vi "VisionV4 2-12-20.vi"(0 "Range (Threshold 1)":cluster{"Lower value":sgl, "Upper value":sgl}={"Lower value"=210.0, "Upper value"=250.0}, 1 "Minimal Score (Shape Matching 1)":dbl=400.0, 2 "Scale Invariance (Shape Matching 1)":bool=TRUE, 3 "Image":T1(plugin-control), 7 "error in":errorcluster) -> (20 "Histogram (Histogram 1)":u32[][](array[numeric]), 21 "Statistics (Histogram 1)":T3 {"Standard  Variation" format="%.2f"; "Mean Value" format="%.2f"; "Maximal Value" format="%.2f"; "Minimal Value" format="%.2f"}, 22 "Number of Matches (Shape Matching 1)":i32, 23 "Shape Report (Shape Matching 1)":T2(array[cluster]) {"Score" format="%.2f"; "Centroid"."y" format="%.2f"; "Centroid"."x" format="%.2f"}, 27 "error out":errorcluster)   [LabVIEW 2019]
uses:
  <vilib>/vision/NI_Vision_Development_Module.lvlib
panel:
  out "Image Out":T1(plugin-control)
  out "Histogram Graph":u32[][](graph)
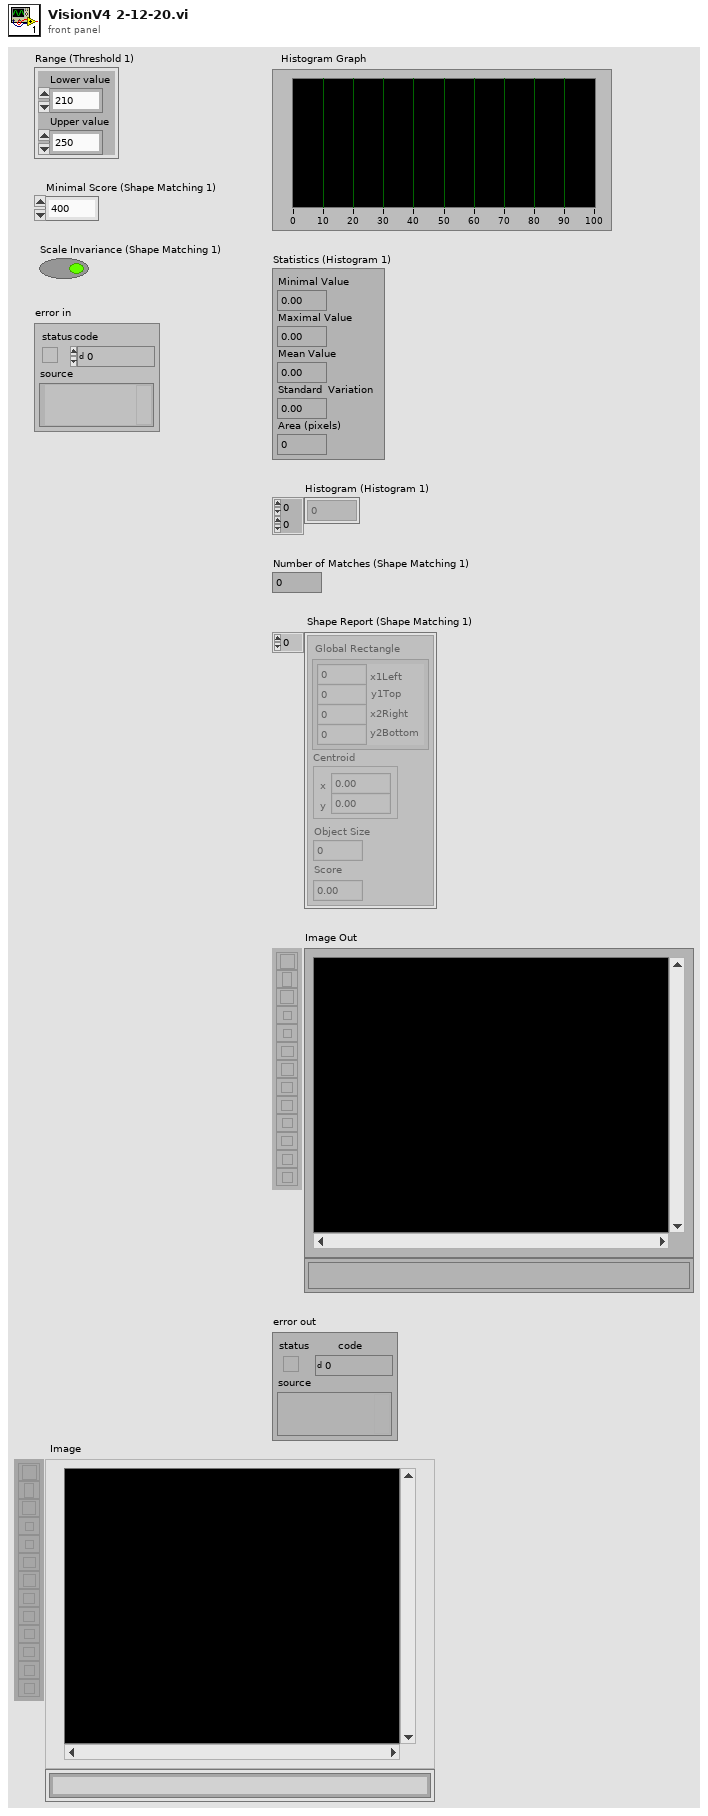
[diagram p1: front panel]
types:
  T1 = typedef "IMAQ Image.ctl" = refnum<image>
  T2 = cluster{"Global Rectangle":cluster{"x1Left":i32, "y1Top":i32, "x2Right":i32, "y2Bottom":i32}, "Centroid":cluster{"x":sgl, "y":sgl}, "Object Size":u32, "Score":dbl}[]
  T3 = cluster{"Minimal Value":sgl, "Maximal Value":sgl, "Mean Value":sgl, "Standard  Variation":sgl, "Area (pixels)":i32}
  T4 = cluster{"Measurement Parameter":i32, "Range Lower Value":dbl, "Range Upper Value":dbl, "Range":bool, "Measurement Type":bool}[]
  T5 = cluster{"Global Rectangle":i32[], "Contours":cluster{"ID":enum32{"External", "Internal"}, "Type":u32, "Coordinates":i32[]}[]}
  T6 = cluster{"histogram":u32[], "Minimal Value":sgl, "Maximal Value":sgl, "Starting Value":sgl, "Interval Width":sgl, "Mean Value":sgl, "Standard  Variation":sgl, "Area (pixels)":i32}
  T7 = typedef "Image Type" = u32
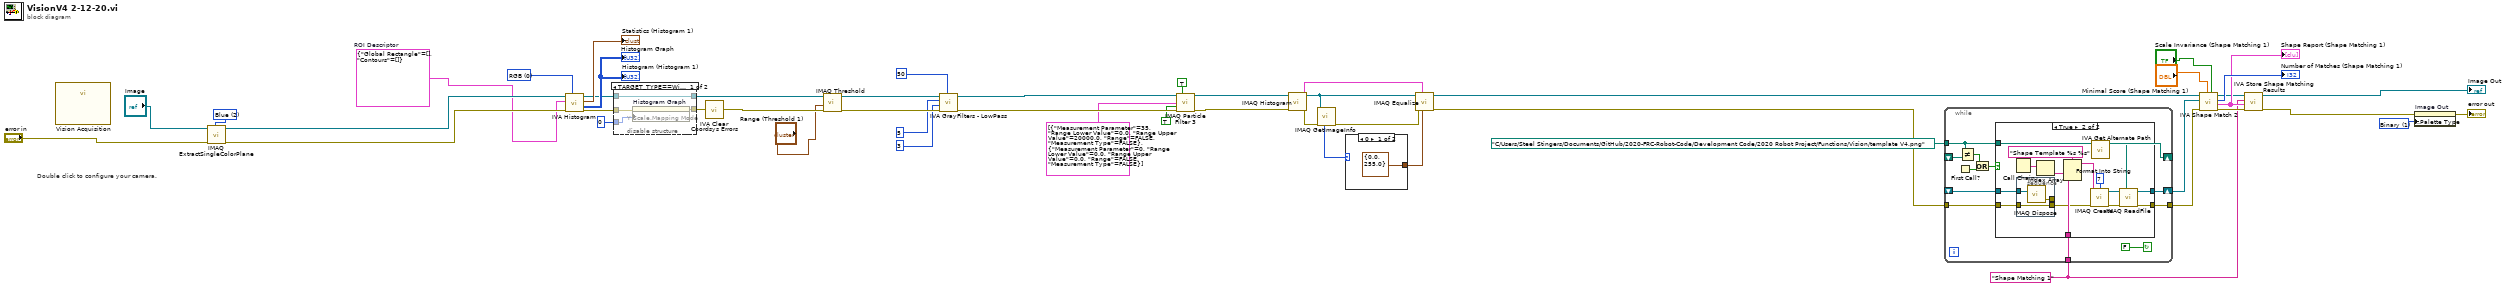
[diagram p0: block diagram]
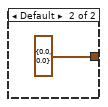
[diagram p3: hidden frame]
diagram:
  w3 = u32 1 items=["Grayscale", "Binary", "Gradient", "Rainbow", "Temperature", "User Defined", "Binary 16 Bit", "Gradient 16 Bit", "Rainbow 16 Bit", "Temperature 16 Bit", "User Defined 16 Bit"] ("Palette Type")
  w6 = "Shape Matching 1" ("Step Name")
  w44 = u16 0 items=["RGB", "HSL", "HSV", "HSI"] ("Color Mode")
  w42 = T5 {"Global Rectangle"=[], "Contours"=[]}  # ROI Descriptor
  w49 = 2 items=["Red", "Green", "Blue", "Hue", "Saturation", "Luminance", "Value", "Intensity"] ("Color Plane")
  # "Double click to configure your camera."
  n1 = call "Vision Acquisition"() -> ()  [unwired: 20 in]
  n2 = call "IMAQ ExtractSingleColorPlane"("Color Plane"=w49, "error in (no error)"="error in", "Image Src"="Image") -> ("error out"=w48:errorcluster, "Image Dst Out"=w47:T1)  [unwired: 1 in, 6 out]
  n3 = call <vilib>:"IVA Histogram.vi"("Color Mode"=w44, "error in (no error)"=w48, "ROI Descriptor"=w42, "Image In"=w47) -> ("error out"=w45:errorcluster, "Histograms"=→"Histogram Graph" →"Histogram (Histogram 1)":u32[][], "Statistics"=→"Statistics (Histogram 1)":T3, "Image Out"=w41:T1)  [unwired: 4 out]
  n4 = disable-structure "Conditional Disable Structure" shown="TARGET_TYPE==Windows" {
    disable-tunnel: w45 -> [w53 w54]
    disable-tunnel: [w52 w54] -> w39
    disable-tunnel: w41 -> [w51 w55]
    disable-tunnel: [w51 w55] -> w36
    disable-tunnel: u8 0 ("Y Scale.Mapping Mode") -> [w50 _]
    frame condition #0 {
      n5 = property on="Histogram Graph" class="WFGraph (strict)"(error in=w53, "Y Scale.Mapping Mode"=w50) -> (error out=w52:errorcluster)  [unwired: 1 in, 1 out]
    }
    frame condition #1 (active) {
    }
  }
  n6 = call <vilib>:"IVA Clear Coordsys Errors.vi"("error in (no error)"=w39) -> ("error out"=w38:errorcluster)  [unwired: 10 in]
  n7 = call "IMAQ Threshold"("error in (no error)"=w38, "Range"="Range (Threshold 1)", "Image Src"=w36) -> ("error out"=w35:errorcluster, "Image Dst Out"=w34:T1)  [unwired: 3 in, 4 out]
  n8 = call <vilib>:"IVA GrayFilters - LowPass.vi"("Tolerance"=50, "error in"=w35, "Filter size Y"=3, "Filter size X"=5, "Image In"=w34) -> ("error out"=w33:errorcluster, "Image Out"=w26:T1)  [unwired: 5 out]
  n9 = call "IMAQ Particle Filter 3"("Image Src"=w26, "Connectivity 4/8 (8)"=TRUE, "Selection Values"=T4 [{"Measurement Parameter"=35, "Range Lower Value"=0.0, "Range Upper Value"=20000.0, "Range"=FALSE, "Measurement Type"=FALSE}, {"Measurement Parameter"=0, "Range Lower Value"=0.0, "Range Upper Value"=0.0, "Range"=FALSE, "Measurement Type"=FALSE}], "Keep/Remove Particles (F)"=TRUE ("Keep/Remove Particles"), "error in (no error)"=w33) -> ("Image Dst Out"=w21:T1, "error out"=w27:errorcluster)  [unwired: 4 in, 5 out]
  n10 = call "IMAQ Histogram"("error in (no error)"=w27, "Image"=w21) -> ("error out"=w20:errorcluster, "Histogram Report"=w23:T6)  [unwired: 3 in, 5 out]
  n11 = call "IMAQ GetImageInfo"("error in (no error)"=w20, "Image"=w21) -> ("error out"=w19:errorcluster, "Image Type"=w22:T7)  [unwired: 8 out]
  n12 = case shown="0" w22 {
    tunnel: [cluster{"Minimum":sgl, "Maximum":sgl} {"Minimum"=0.0, "Maximum"=255.0} ("Range") cluster{"Minimum":sgl, "Maximum":sgl} {"Minimum"=0.0, "Maximum"=0.0} ("Range")] -> w18
    frame 0 {
    }
    frame Default {
    }
  }
  n13 = call "IMAQ Equalize"("Range"=w18, "Histogram Report"=w23, "error in (no error)"=w19, "Image Src"=w21) -> ("error out"=w24:errorcluster, "Image Dst Out"=w14:T1)  [unwired: 2 in, 4 out]
  n14 = while {
    shift-right: [w68] -> w7
    shift-left: _ -> [w67]
    tunnel: [w65] -> w8
    tunnel: w24 -> [w64]
    tunnel: path "C:/Users/Steel Stingers/Documents/GitHub/2020-FRC-Robot-Code/Development Code/2020 Robot Project/Functions/Vision/template V4.png" ("Template Path") -> [w62]
    tunnel: w6 -> [w63]
    shift-right: [w62] -> _
    shift-left: _ -> [w61]
    stop <- FALSE continue-if-true
    n15 = First Call?() -> (First Call?: T/F=w60:bool)
    n16 = Not Equal?(x=w62, y=w61) -> (x != y?=w59:bool)
    n17 = Or(x=w59, y=w60) -> (x .or. y?=w58:bool)
    n18 = case shown="True" w58 {
      tunnel: [w70 w82] -> w68
      tunnel: w67 -> [w70 w73]
      tunnel: [w69 w80] -> w65
      tunnel: w64 -> [w69 w72]
      tunnel: w62 -> [_ w75]
      tunnel: w63 -> [_ w76]
      frame False {
      }
      frame True {
        n19 = Call Chain() -> (call chain=w78:string[])
        n20 = stacked-sequence {
          tunnel: w73 -> [w88]
          tunnel: w72 -> [w87]
          tunnel: [w87] -> w71
          tunnel: [w86] -> _
          frame #0 {
            n21 = call "IMAQ Dispose"("Image"=w88) -> ("error out"=w86:errorcluster)  [unwired: 2 in, 3 out]
          }
        }
        n22 = Index Array(array=w78) -> (element=w77:string)  [unwired: 1 in]
        n23 = Format Into String(format string="Shape Template %s %s" ("Image Name"), w77, w76) -> (resulting string=w85:string)  [unwired: 2 in, 1 out]
        n24 = call "IMAQ Create"("Border Size"=7, "Image Name"=w85, "error in (no error)"=w71) -> ("New Image"=w83:T1, "error out"=w81:errorcluster)  [unwired: 1 in, 1 out]
        n25 = call <vilib>:"IVA Get Alternate Path.vi"("Path In"=w75) -> ("Path Out"=w74:path)  [unwired: 10 out]
        n26 = call "IMAQ ReadFile"("File Path"=w74, "error in (no error)"=w81, "Image"=w83) -> ("error out"=w80:errorcluster, "Image Out"=w82:T1)  [unwired: 2 in, 5 out]
      }
    }
  }
  n27 = call <vilib>:"IVA Shape Match 2.vi"("Scale Invariance"="Scale Invariance (Shape Matching 1)", "Minimal Score"="Minimal Score (Shape Matching 1)", "error in (no error)"=w8, "Template"=w7, "Image Src"=w14) -> ("error out"=w13:errorcluster, "Shape Report"=w11:T2, "Number of Matches"=→"Number of Matches (Shape Matching 1)":i32, "Image Out"=w10:T1)  [unwired: 3 out]
  "Shape Report (Shape Matching 1)" <- w11
  n28 = call <vilib>:"IVA Store Shape Matching Results.vi"("error in (no error)"=w13, "Shape Report"=w11, "Step Name"=w6, "Image in"=w10) -> ("error out"=w12:errorcluster, "Image dup"=→"Image Out":T1)  [unwired: 6 out]
  n29 = property on="Image Out" class="ImageControl"(error in=w12, "Palette:Palette Type"=w3) -> (error out=→"error out":errorcluster)  [unwired: 1 in, 1 out]
